vi "Validate_Destinations.vi"(8 "error in (no error)":errorcluster, 11 "Installer in":refnum<class "Installer.lvclass">) -> (0 "error out":errorcluster, 3 "Installer out":refnum<class "Installer.lvclass">)   [LabVIEW 2020, in "Installer.lvclass"]
uses:
  <vilib>/AppBuilder/IB_Classes/Installer/Installer.lvclass
  <vilib>/AppBuilder/IB_Classes/Installer/Installer.lvclass/Installer.ctl
  <vilib>/AppBuilder/IB_Classes/Destination/IB_Destination.lvclass
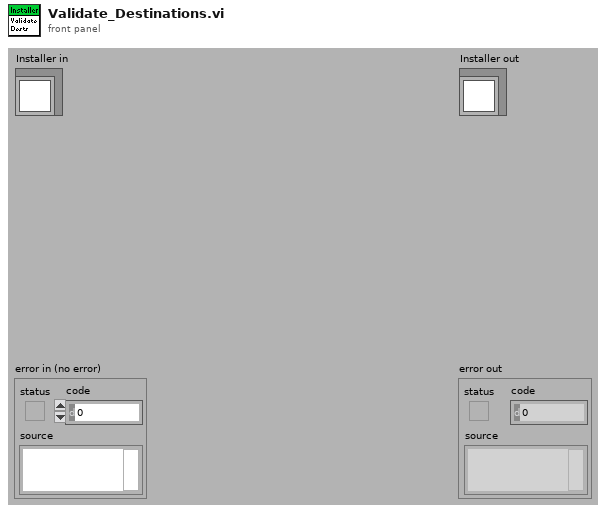
[diagram p1: front panel]
types:
  T1 = typedef "IB_Destination.ctl" = cluster{"name":string, "unlock":bool, "parentTag":string, "destTag":string, "eng_installPath":string}
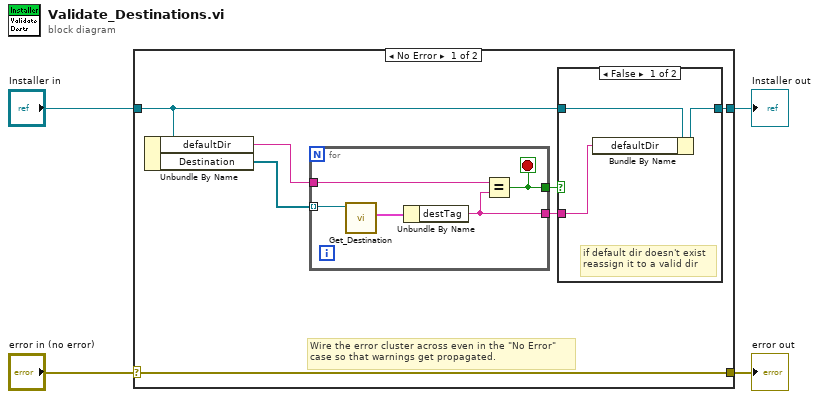
[diagram p0: block diagram]
diagram:
  n1 = case shown="No Error" "error in (no error)" {
    selector: "error in (no error)" -> [w11 w22]
    tunnel: [w11 w22] -> w3
    tunnel: [w7 w21] -> w1
    tunnel: "Installer in" -> [w8 w21]
    frame No Error {
      # "Wire the error cluster across even in the \"No Error\"\ncase so that warnings get propagated."
      n2 = Unbundle By Name(w8) -> ("defaultDir"=w9:string, "Destination"=w10:refnum<class "IB_Destination.lvclass">[])
      n3 = for {
        tunnel: w10 -> [w20] mode=indexing
        tunnel: w9 -> [w18]
        tunnel: [w17] -> w5
        tunnel: [w16] -> w6
        stop <- w16 stop-if-true
        n4 = call <vilib>:"Get_Destination.vi"("IB_Destination in"=w20) -> ("data"=w19:T1)  [unwired: 8 in, 2 out]
        n5 = Unbundle By Name(w19) -> ("destTag"=w17:string)
        n6 = Equal?(x=w18, y=w17) -> (x = y?=w16:bool)
      }
      n7 = case shown="False" w6 {
        tunnel: w8 -> [w14 w15]
        tunnel: [w13 w15] -> w7
        tunnel: w5 -> [w12 _]
        frame False {
          # "if default dir doesn't exist\nreassign it to a valid dir"
          n8 = Bundle By Name(cluster=w14, "defaultDir"=w12) -> (w13:refnum<class "Installer.lvclass">)
        }
        frame True {
        }
      }
    }
    frame Error {
    }
  }
  "error out" <- w3
  "Installer out" <- w1
